vi "SetupStriptest.vi"(3 "Probe Card Channels":i32=32) -> (1 "Continue?":bool)   [LabVIEW 2013]
uses:
  ProbePlan/ProbePlanParams.vi
  general_VIs/globals/QC_RunInformation.vi
  general_VIs/globals/QC_MeasurementSetup.vi
panel:
  in  "Sensor Bias":dbl=-150.0
  out "Instructions:":string="- configure Arduino edgesense; optional testing of edgesense                                        - define probing range\n- select LCR meter, bias, and IV supply; configure if necessary                                         - adjust measurement parameters\n- select operator                                                                                                          - select tests included"
  in  "Bias Supply":u16(ring) items=["Keithley 487", "Keithley 6517", "Keithley 236/237", "Keithley 2410"]
  in  "Test Button":bool
  in  "Resistance Y/N":bool=TRUE
  in  "Capacitance Y/N":bool=TRUE
  in  "Pinholes Y/N":bool=TRUE
  in  "High Step":i32=1000
  in  "Base Step":i32=1000
  in  "High Ramp":dbl=100.0
  in  "Base Ramp":dbl=10.0
  in  "High V":dbl=100.0
  in  "Base V":dbl=10.0
  in  "Quit":bool
  in  "Continue":bool
  in  "Settings Button":bool
  in  "T/RH Readout":enum16{"Arduino Uno", "Nothing"}(ring)
  in  "LCR meter:":u16(ring) items=["WK 6440B", "WK 6425", "HP 4263B"]
  in  "IV Supply:":u16(ring)=3 items=["Keithley 487", "Keithley 6517", "Keithley 236/237", "Keithley 2410"]
  in  "Operator:":u32(ring) items=["Saevar", "Maurice", "Rick", "Dave", "Bart", "Miguel", "Christoph", "Other..."]
  out "DataBase Serial No.:":string
  out "Manufacturer:":string
  out "Device Category:":string
  out "Manufacturer Serial No.:":string
  out "Region4":string
  out "Region3":string
  out "Region2":string
  out "Region":string
  in  "From4":u16(ring)
  in  "From3":u16(ring)
  in  "From2":u16(ring)
  in  "From":u16(ring)
  in  "To4":u16(ring)
  in  "To3":u16(ring)
  in  "To2":u16(ring)
  in  "To":u16(ring)
  in  "Enable4":bool
  in  "Enable3":bool
  in  "Enable2":bool
  in  "Enable1":bool
  # "Setup Striptest"
  # "Define Probe Range"
  # "Measurement Parameters"
  # "Volts"
  # "Base Voltage Settings"
  # "High Voltage Settings"
  # "Volts"
  # "Volts"
  # "Volts/step"
  # "Volts/step"
  # "millisec"
  # "millisec"
  # "DUT & Test Description"
  # "Tests Included"
  # "Hardware"
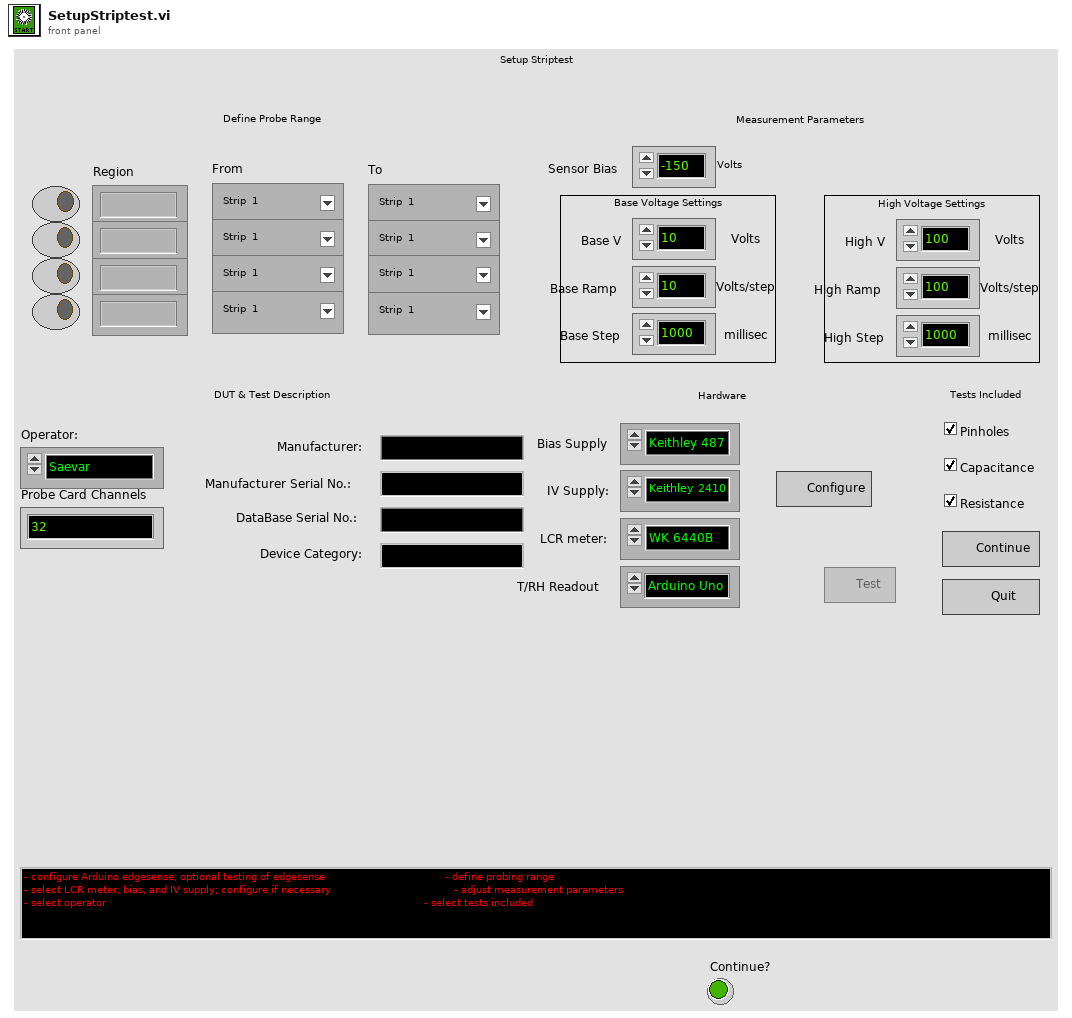
[diagram p1: front panel]
types:
  T1 = cluster{"Strip Number OUT":i32, "X0":i32, "Y0":i32, "X1":i32, "Y1":i32, "Xref":dbl, "Yref":dbl, "ProbePlan type":u32, "Inner pads offset":ext, "Outer pads offset":ext, "l_inner":ext, "l_outer":ext, "strip numbering":u16, "Device Orientation":ext, "Stagger offset":i32, "Yoffset":dbl, "Strip pitch":dbl, "Fiducail separation":dbl, "Radius":ext, "Relative strip angles":dbl, "Probeplan description":string, "ProbePlan array":cluster{"Region":string, "ProbePoints":cluster{"X":dbl, "Y":dbl, "Label":string, "CardViable?":bool}[]}[], "Test ProbePoints":cluster{"Regions Enabled":bool[], "From index":u32[], "To index":u32[]}}
  T2 = cluster{"Region":string, "ProbePoints":cluster{"X":dbl, "Y":dbl, "Label":string, "CardViable?":bool}[]}[]
  T3 = cluster{"Sensor Serial No.:":string, "Wafer Serial No.:":string, "Batch:":string, "Manufacturer:":string, "Device Category:":string, "Database Serial No.:":string, "Date Initiated:":string, "Time Initiated:":string, "Test":string, "Instruments used:":string, "Probeplan used:":string, "End of Run comment:":string, "User:":string}
  T4 = cluster{"Bias Supply":refnum<class "SupplyControl.lvclass">, "SMU":refnum<class "SupplyControl.lvclass">, "LCR":refnum<class "LCRControl.lvclass">, "Probe Card Channels":i32, "Bias Voltage [V]":dbl, "First strip":i32, "Last strip":i32, "Base Voltage [V]":dbl, "Base Ramp Step [V]":dbl, "Base Ramp Interval [ms]":u32, "High Voltage [V]":dbl, "High Ramp Step [V]":dbl, "High Ramp Interval [ms]":u32, "Single Needle":bool, "Temperature Readout":enum16{"Read Arduino", "Enter manually"}, "Arduino":refnum<class "ArduinoControl.lvclass">, "Fraction of good strips [%]":dbl, "ProbeStation":refnum<class "ProbeStationControl.lvclass">, "AC frequency [Hz]":i32, "Switching":refnum<class "Switching.lvclass">, "Matrix used?":bool, "Matrix X Channels":cluster{"Bias Supply / SMU LO":i32, "Bias Supply / SMU HI":i32, "CV Box LO":i32, "CV Box HI":i32, "CV Box LO IN":i32, "CV Box HI IN":i32, "Volt meter LO":i32, "Volt meter HI":i32, "Mux1 C1":i32, "Mux1 C2":i32, "Mux2 C1":i32, "Mux2 C2":i32}, "Pinholes Y/N":bool, "Capacitance Y/N":bool, "Resistance Y/N":bool}
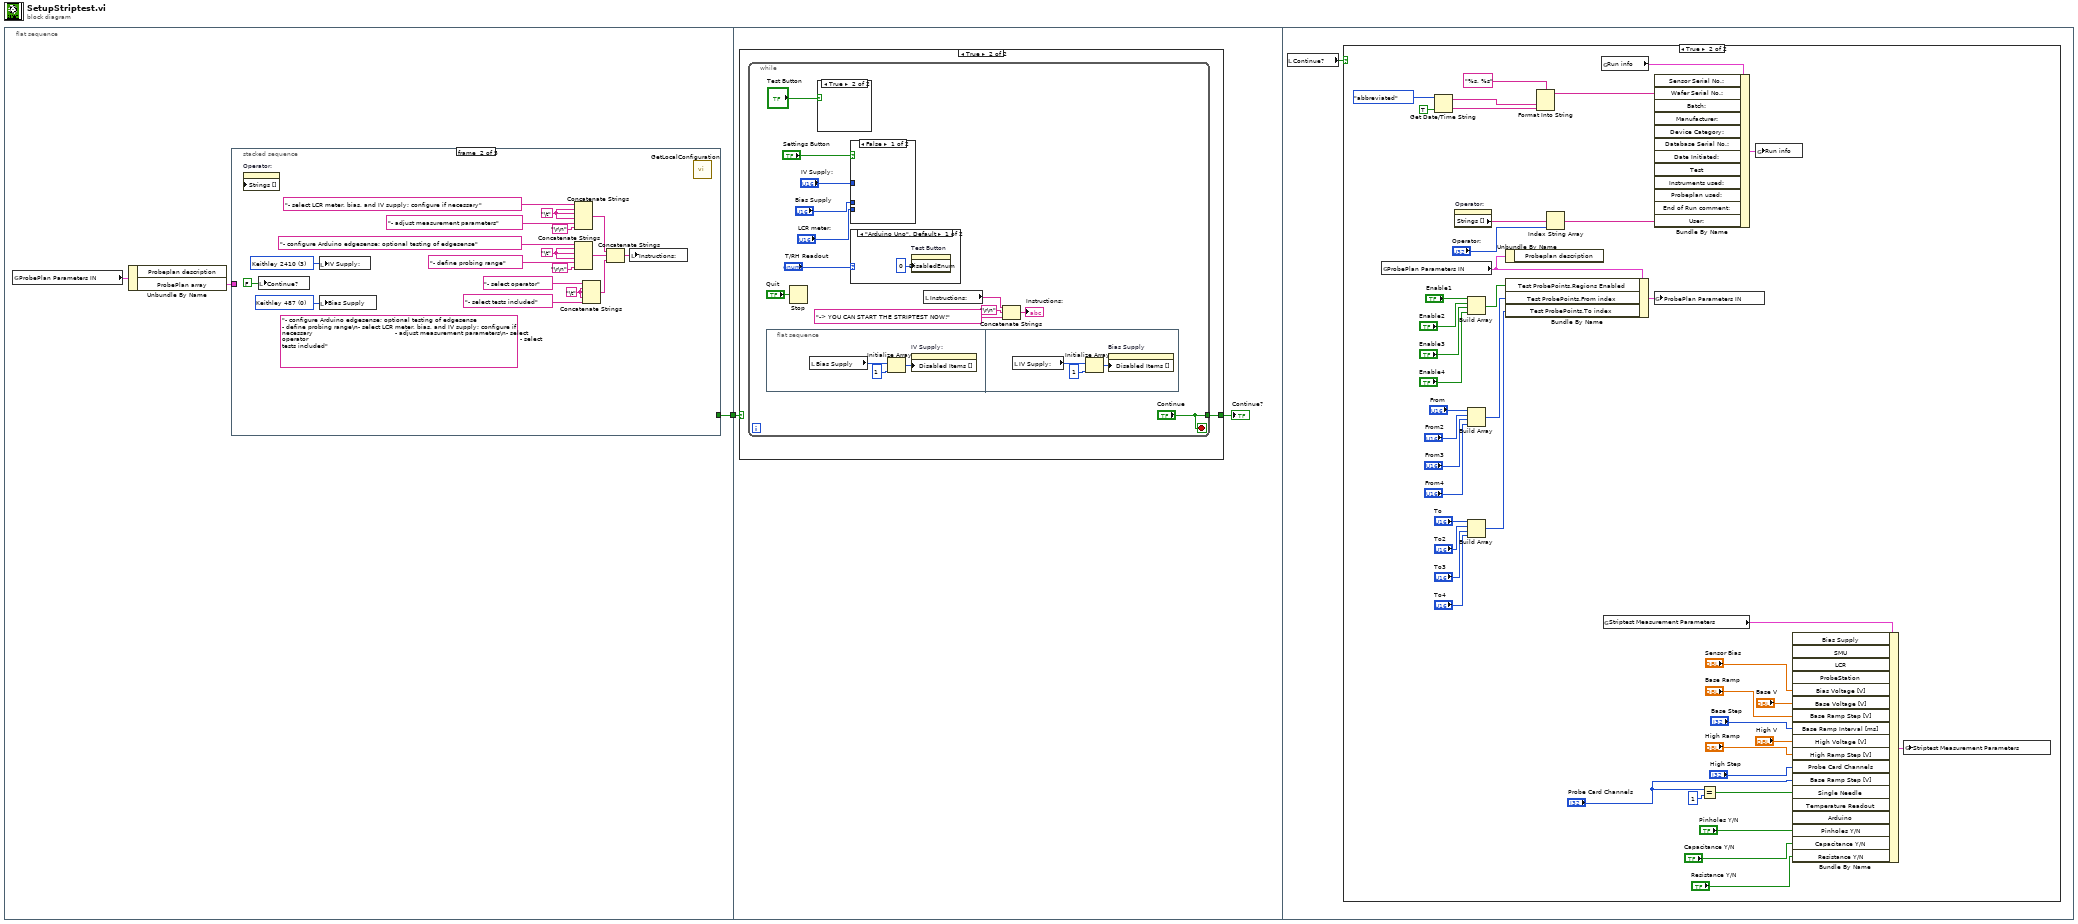
[diagram p0: block diagram]
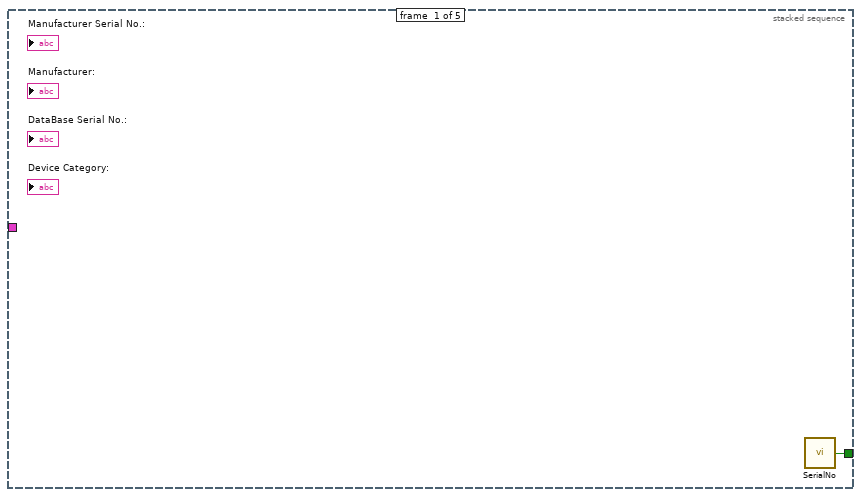
[diagram p2: hidden frame]
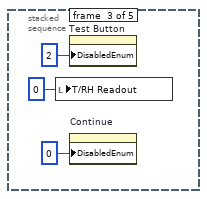
[diagram p3: hidden frame]
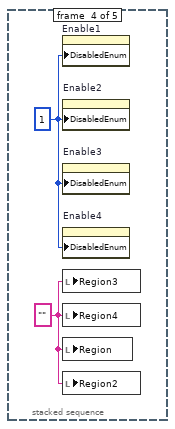
[diagram p4: hidden frame]
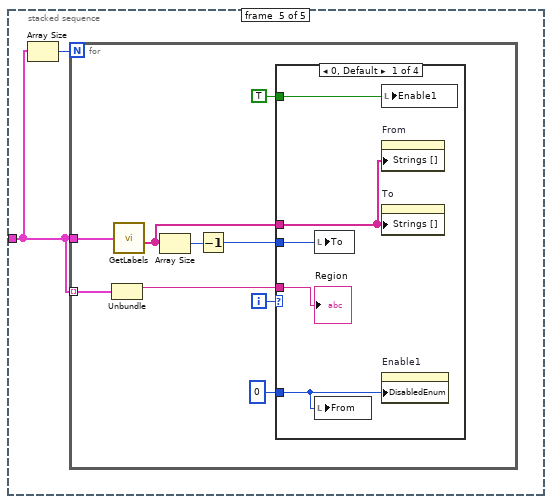
[diagram p5: hidden frame]
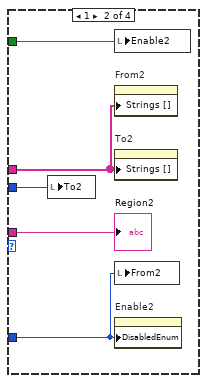
[diagram p6: hidden frame]
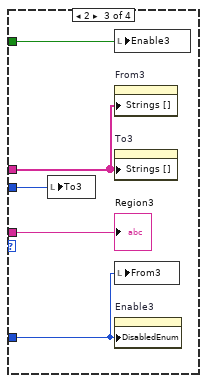
[diagram p7: hidden frame]
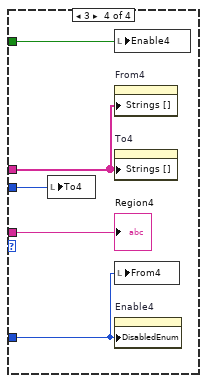
[diagram p8: hidden frame]
diagram:
  n1 = flat-sequence {
    tunnel: [w2] -> w1
    tunnel: w1 -> [w60]
    frame #0 {
      n2 = global read "ProbePlanParams.vi" "ProbePlan Parameters IN"() -> (w4:T1)
      n3 = Unbundle By Name(w4) -> ("ProbePlan array"=w3:T2)  [unwired: 1 out]
      n4 = stacked-sequence {
        tunnel: w3 -> [_ _ _ _ w29]
        tunnel: [w5 _ _ _ _] -> w2
        frame #0 {
          n5 = call "SerialNo.vi"() -> ("Continue?"=w5:bool)  [unwired: 5 in]
        }
        frame #1 {
          w14 = "\t"
          w16 = "\t"
          w20 = "\t"
          (unwired) "- configure Arduino edgesense; optional testing of edgesense                                        - define probing range\n- select LCR meter, bias, and IV supply; configure if necessary                                         - adjust measurement parameters\n- select operator                                                                                                          - select tests included" ("Instructions:")
          w21 = u16 0 items=["Keithley 487", "Keithley 6517", "Keithley 236/237", "Keithley 2410"] ("Supply:")
          w22 = u16 3 items=["Keithley 487", "Keithley 6517", "Keithley 236/237", "Keithley 2410"] ("Supply:")
          n6 = property on="Operator:" class="Ring (strict)" props=["Strings []"]() -> ()  [unwired: 3 in, 2 out]
          n7 = local write "Continue?"(FALSE ("Continue?")) -> ()
          n8 = local write "IV Supply:"(w22) -> ()
          n9 = local write "Bias Supply"(w21) -> ()
          n10 = Concatenate Strings("- select LCR meter, bias, and IV supply; configure if necessary", w16, w16, w16, "- adjust measurement parameters", "\r\n") -> (w9:string)
          n11 = Concatenate Strings("- configure Arduino edgesense; optional testing of edgesense", w20, w20, w20, "- define probing range", "\r\n") -> (w10:string)
          n12 = Concatenate Strings("- select operator", w14, w14, w14, "- select tests included") -> (w11:string)
          n13 = Concatenate Strings(w9, w10, w11) -> (w8:string)
          n14 = local write "Instructions:"(w8) -> ()
          n15 = call "GetLocalConfiguration.vi"() -> ()  [unwired: 3 in, 1 out]
        }
        frame #2 {
          n16 = local write "T/RH Readout"(0) -> ()
          n17 = property on="Test Button" class="Bool"("DisabledEnum"=2) -> ()  [unwired: 2 in, 2 out]
          n18 = property on="Continue" class="Bool"("DisabledEnum"=u8 0 ("Disabled")) -> ()  [unwired: 2 in, 2 out]
        }
        frame #3 {
          w28 = "" ("Region")
          w27 = u8 1 ("Disabled")
          n19 = property on="Enable1" class="Bool (strict)"("DisabledEnum"=w27) -> ()  [unwired: 2 in, 2 out]
          n20 = property on="Enable2" class="Bool (strict)"("DisabledEnum"=w27) -> ()  [unwired: 2 in, 2 out]
          n21 = property on="Enable3" class="Bool (strict)"("DisabledEnum"=w27) -> ()  [unwired: 2 in, 2 out]
          n22 = property on="Enable4" class="Bool (strict)"("DisabledEnum"=w27) -> ()  [unwired: 2 in, 2 out]
          n23 = local write "Region3"(w28) -> ()
          n24 = local write "Region4"(w28) -> ()
          n25 = local write "Region"(w28) -> ()
          n26 = local write "Region2"(w28) -> ()
        }
        frame #4 {
          n27 = Array Size(array=w29) -> (size(s)=w30:i32)
          n28 = for {
            N: w30 -> [_]
            tunnel: w29 -> [w32]
            tunnel: w29 -> [w36] mode=indexing
            i -> [w39]
            n29 = Unbundle(w36) -> ("Region"=w35:string)  [unwired: 1 out]
            n30 = call "GetLabels.vi"("Array"=w32) -> ("Strip Labels"=w31:string[])  [unwired: 3 out]
            n31 = Array Size(array=w31) -> (size(s)=w34:i32)
            n32 = Decrement(x=w34) -> (x-1=w33:i32)
            n33 = case shown="0, Default" w39 {
              tunnel: TRUE -> [w44 w48 w54 w59]
              tunnel: 0 -> [w40 w45 w50 w55]
              tunnel: w35 -> [w42 w47 w52 w57]
              tunnel: w31 -> [w41 w46 w51 w56]
              tunnel: w33 -> [w43 w49 w53 w58]
              frame 0, Default {
                n34 = local write "To"(w43) -> ()
                n35 = local write "From"(w40) -> ()
                n36 = local write "Enable1"(w44) -> ()
                n37 = property on="From" class="Ring (strict)"("Strings []"=w41) -> ()  [unwired: 2 in, 2 out]
                n38 = property on="To" class="Ring (strict)"("Strings []"=w41) -> ()  [unwired: 2 in, 2 out]
                n39 = property on="Enable1" class="Bool (strict)"("DisabledEnum"=w40) -> ()  [unwired: 2 in, 2 out]
                "Region" <- w42
              }
              frame 1 {
                n40 = local write "To2"(w49) -> ()
                n41 = local write "Enable2"(w48) -> ()
                n42 = property on="From2" class="Ring (strict)"("Strings []"=w46) -> ()  [unwired: 2 in, 2 out]
                n43 = property on="To2" class="Ring (strict)"("Strings []"=w46) -> ()  [unwired: 2 in, 2 out]
                n44 = local write "From2"(w45) -> ()
                n45 = property on="Enable2" class="Bool (strict)"("DisabledEnum"=w45) -> ()  [unwired: 2 in, 2 out]
                "Region2" <- w47
              }
              frame 2 {
                n46 = local write "To3"(w53) -> ()
                n47 = local write "Enable3"(w54) -> ()
                n48 = property on="From3" class="Ring (strict)"("Strings []"=w51) -> ()  [unwired: 2 in, 2 out]
                n49 = property on="To3" class="Ring (strict)"("Strings []"=w51) -> ()  [unwired: 2 in, 2 out]
                n50 = local write "From3"(w50) -> ()
                n51 = property on="Enable3" class="Bool (strict)"("DisabledEnum"=w50) -> ()  [unwired: 2 in, 2 out]
                "Region3" <- w52
              }
              frame 3 {
                n52 = local write "To4"(w58) -> ()
                n53 = local write "Enable4"(w59) -> ()
                n54 = property on="From4" class="Ring (strict)"("Strings []"=w56) -> ()  [unwired: 2 in, 2 out]
                n55 = property on="To4" class="Ring (strict)"("Strings []"=w56) -> ()  [unwired: 2 in, 2 out]
                n56 = local write "From4"(w55) -> ()
                n57 = property on="Enable4" class="Bool (strict)"("DisabledEnum"=w55) -> ()  [unwired: 2 in, 2 out]
                "Region4" <- w57
              }
            }
          }
        }
      }
    }
    frame #1 {
      n58 = case shown="True" w60 {
        selector: w60 -> [w62 _]
        tunnel: [w62 w63] -> w61
        frame False {
        }
        frame True {
          n59 = while {
            tunnel: ["Continue"] -> w63
            stop <- "Continue" stop-if-true
            n60 = flat-sequence {
              frame #0 {
                n61 = local read "Bias Supply"() -> (w77:u16)
                n62 = Initialize Array(w77, 1) -> (w78:u16[])
                n63 = property on="IV Supply:" class="Ring (strict)"("Disabled Items []"=w78) -> ()  [unwired: 2 in, 2 out]
              }
              frame #1 {
                n64 = local read "IV Supply:"() -> (w82:u16)
                n65 = Initialize Array(w82, 1) -> (w80:u16[])
                n66 = property on="Bias Supply" class="Ring (strict)"("Disabled Items []"=w80) -> ()  [unwired: 2 in, 2 out]
              }
            }
            n67 = Stop(stop? (T)="Quit") -> ()
            n68 = case shown="True" "Test Button" {
              frame False {
              }
              frame True {
              }
            }
            n69 = case shown="False" "Settings Button" {
              tunnel: "IV Supply:" -> [_ _]
              tunnel: "LCR meter:" -> [_ _]
              tunnel: "Bias Supply" -> [_ _]
              frame False {
              }
              frame True {
              }
            }
            n70 = case shown="\"Arduino Uno\", Default" "T/RH Readout" {
              frame "Arduino Uno", Default {
                n71 = property on="Test Button" class="Bool"("DisabledEnum"=0) -> ()  [unwired: 2 in, 2 out]
              }
              frame "Nothing" {
              }
            }
            n72 = local read "Instructions:"() -> (w66:string)
            n73 = Concatenate Strings(w66, "\r\n", "-> YOU CAN START THE STRIPTEST NOW!") -> (→"Instructions:":string)
          }
        }
      }
      "Continue?" <- w61
    }
    frame #2 {
      n74 = local read "Continue?"() -> (w83:bool)
      n75 = case shown="True" w83 {
        frame False {
        }
        frame True {
          n76 = global read "ProbePlanParams.vi" "ProbePlan Parameters IN"() -> (w103:T1)
          n77 = Get Date/Time String(date format (0)=enum16{"short", "long", "abbreviated"}."abbreviated", want seconds? (F)=TRUE) -> (date string=w99:string, time string=w98:string)  [unwired: 1 in]
          n78 = property on="Operator:" class="Ring (strict)"() -> ("Strings []"=w104:string[])  [unwired: 2 in, 2 out]
          n79 = Build Array("Enable1", "Enable2", "Enable3", "Enable4") -> (w112:bool[])
          n80 = Build Array("From", "From2", "From3", "From4") -> (w113:u16[])
          n81 = Build Array("To", "To2", "To3", "To4") -> (w114:u16[])
          n82 = Unbundle By Name(w103) -> ()  [unwired: 1 out]
          n83 = Bundle By Name(cluster=w103, "Test ProbePoints.Regions Enabled"=w112, "Test ProbePoints.From index"=w113, "Test ProbePoints.To index"=w114) -> (w111:T1)
          n84 = Format Into String(format string="%s, %s", w99, w98) -> (resulting string=w97:string)  [unwired: 2 in, 1 out]
          n85 = Index String Array(1:"Operator:", 2:w104) -> (0:w90:string)  [unwired: 1 in]
          n86 = global read "QC_RunInformation.vi" "Run info"() -> (w92:T3)
          n87 = global read "QC_MeasurementSetup.vi" "Striptest Measurement Parameters"() -> (w85:T4)
          n88 = Bundle By Name(cluster=w92, "Wafer Serial No.:"=w97, "User:"=w90) -> (w93:T3)  [unwired: 10 in]
          n89 = global write "ProbePlanParams.vi" "ProbePlan Parameters IN"(w111) -> ()
          n90 = Equal?(x="Probe Card Channels", y=1) -> (x = y?=w94:bool)
          n91 = global write "QC_RunInformation.vi" "Run info"(w93) -> ()
          n92 = Bundle By Name(cluster=w85, "Bias Voltage [V]"="Sensor Bias", "Base Voltage [V]"="Base V", "Base Ramp Step [V]"="Base Ramp", "Base Ramp Interval [ms]"="Base Step", "High Voltage [V]"="High V", "High Ramp Step [V]"="High Ramp", "Probe Card Channels"="High Step", "Base Ramp Step [V]"="Probe Card Channels", "Single Needle"=w94, "Pinholes Y/N"="Pinholes Y/N", "Capacitance Y/N"="Capacitance Y/N", "Resistance Y/N"="Resistance Y/N") -> (w91:T4)  [unwired: 6 in]
          n93 = global write "QC_MeasurementSetup.vi" "Striptest Measurement Parameters"(w91) -> ()
        }
      }
    }
  }
